vi "Cluster to Variant Array.vi"(8 "error in (no error)":errorcluster, 11 "Variant":variant) -> (0 "error out":errorcluster, 1 "Values":variant[](array[variant]), 2 "Names":string[](array[string]))   [LabVIEW 2017]
uses:
  <vilib>/Utility/Data Type/NI_Data Type.lvlib
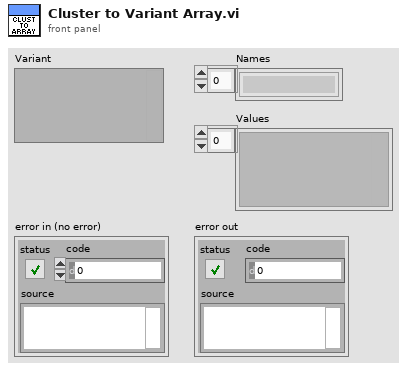
[diagram p1: front panel]
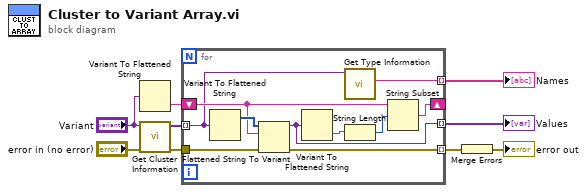
[diagram p0: block diagram]
diagram:
  n1 = Variant To Flattened String(Variant="Variant") -> (data string=w2:string)  [unwired: 1 out]
  n2 = call <vilib>:"Get Cluster Information.vi"("error in (no error)"="error in (no error)", "Variant"="Variant") -> ("error out"=w4:errorcluster, "Cluster Elements"=w3:variant[])  [unwired: 8 in]
  n3 = for {
    tunnel: w3 -> [w11] mode=indexing
    tunnel: [w18] -> w6 mode=indexing
    shift-right: [w14] -> _
    shift-left: w2 -> [w17]
    tunnel: w4 -> [w13]
    tunnel: [w12] -> w5 mode=indexing
    tunnel: [w10] -> w1 mode=indexing
    n4 = Variant To Flattened String(Variant=w11) -> (1:w19:i16[])  [unwired: 1 out]
    n5 = Flattened String To Variant(4:w13, 6:w17, 7:w19) -> (0:w12:errorcluster, 3:w18:variant)
    n6 = Variant To Flattened String(Variant=w18) -> (data string=w16:string)  [unwired: 1 out]
    n7 = call <vilib>:"Get Type Information.vi"("Variant"=w11) -> ("Name"=w10:string)  [unwired: 6 in, 4 out]
    n8 = String Length(string=w16) -> (length=w15:i32)
    n9 = String Subset(string=w17, offset (0)=w15) -> (substring=w14:string)  [unwired: 1 in]
  }
  "Values" <- w6
  "Names" <- w1
  n10 = Merge Errors(w5) -> (→"error out":errorcluster)
